vi "Close.vi"(8 "error in (no error)":errorcluster caption="entrée d'erreur (pas d'erreur)", 11 "Class LED Analyser in":refnum<class "Class LED Analyser FEASA.lvclass">) -> (0 "error out":errorcluster caption="sortie d'erreur", 3 "Class LED Analyser Out":refnum<class "Class LED Analyser FEASA.lvclass">)   [LabVIEW 2020, in "Library Instrument & Equipement.lvlib" / "Library LED Analyser.lvlib" / "Class LED Analyser FEASA.lvclass"]
uses:
  Class LED Analyser FEASA.lvclass
  C:/Users/ngarcin/OneDrive - Altyor/Standard TB/Class/LED Analyser/Class Led Analyser (Default)/Class LED Analyser (Default).lvclass
  Class LED Analyser FEASA.lvclass/Class LED Analyser FEASA.ctl
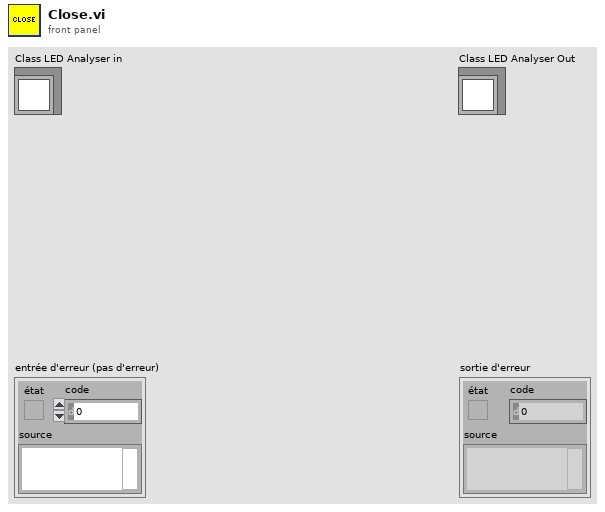
[diagram p1: front panel]
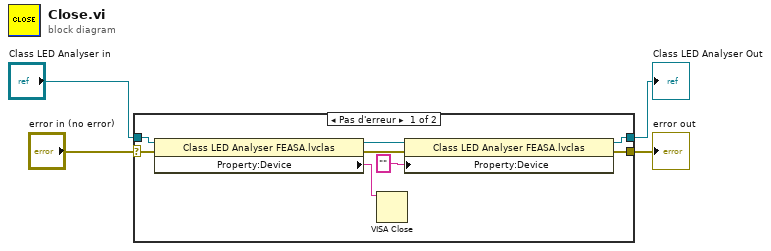
[diagram p0: block diagram]
diagram:
  n1 = case shown="Pas d'erreur" "error in (no error)" {
    selector: "error in (no error)" -> [w11 w14]
    tunnel: [w5 w14] -> w3
    tunnel: [w7 w13] -> w1
    tunnel: "Class LED Analyser in" -> [w12 w13]
    frame No Error {
      n2 = property class="Class LED Analyser FEASA.lvclas"(reference=w12, error in=w11) -> (reference out=w8:refnum<class "Class LED Analyser FEASA.lvclass">, error out=w9:errorcluster, "Property:Device"=w10:string)
      n3 = VISA Close(VISA resource name=w10) -> ()  [unwired: 1 in, 1 out]
      n4 = property class="Class LED Analyser FEASA.lvclas"(reference=w8, error in=w9, "Property:Device"="" ("Device")) -> (reference out=w7:refnum<class "Class LED Analyser FEASA.lvclass">, error out=w5:errorcluster)
    }
    frame Error {
    }
  }
  "error out" <- w3
  "Class LED Analyser Out" <- w1
